vi "SetExternalInterface.vi"(8 "ErrorIn":errorcluster, 10 "ObjectName":string) -> (0 "ErrorOut":errorcluster)   [LabVIEW 2021]
uses:
  Interface_TAF_ITAFObject/ITAFObject/ITAFObject.lvclass
  Interface_TAF_IApplicationConfiguration/IApplicationConfiguration/IApplicationConfiguration.lvclass
  Application.lvclass
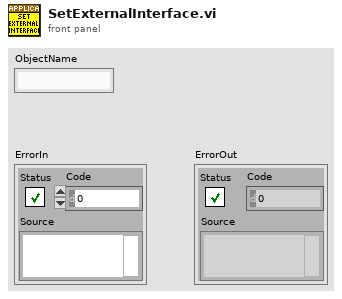
[diagram p1: front panel]
types:
  T1 = typedef "Application.lvclass/ObjectAttributes.ctl" = cluster{"Objects":variant, "BasePath":path, "Application":refnum<class "Application.lvclass">}
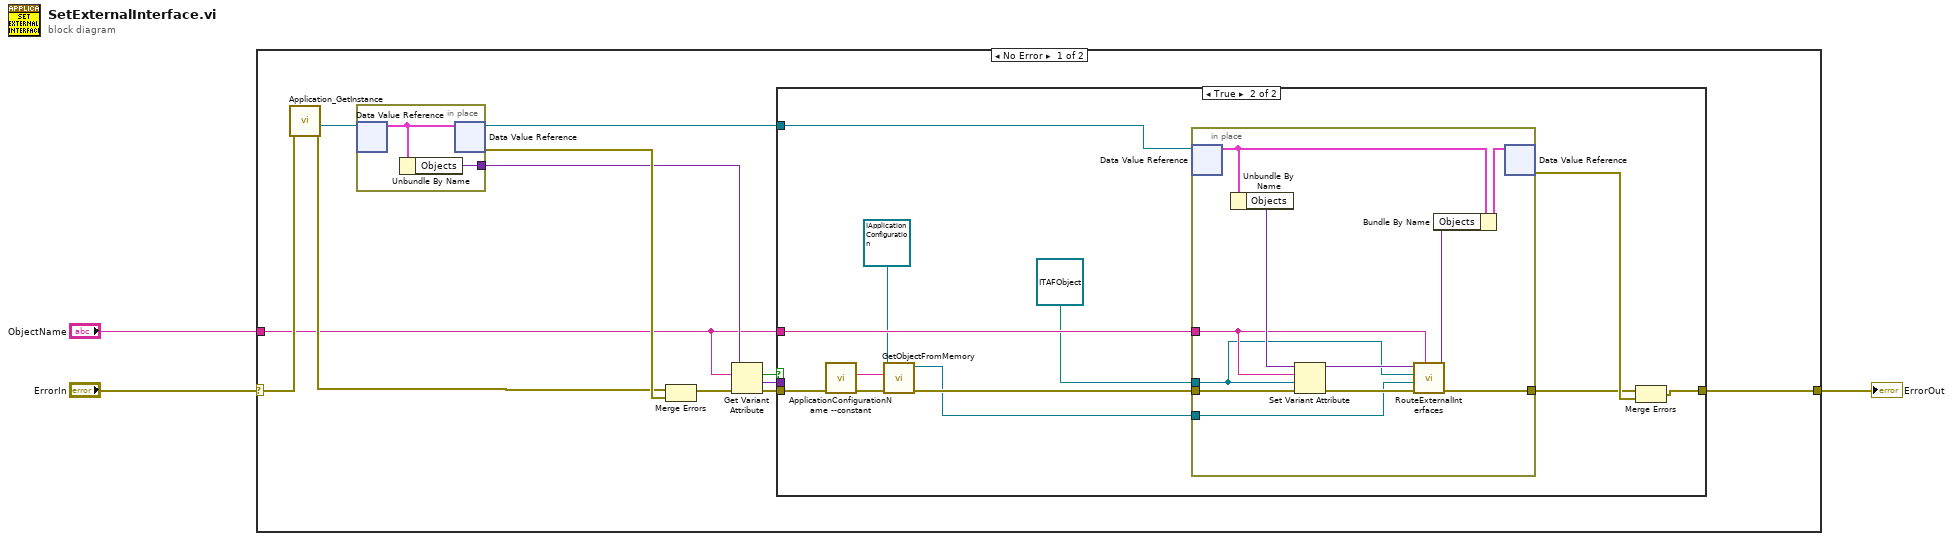
[diagram p0: block diagram]
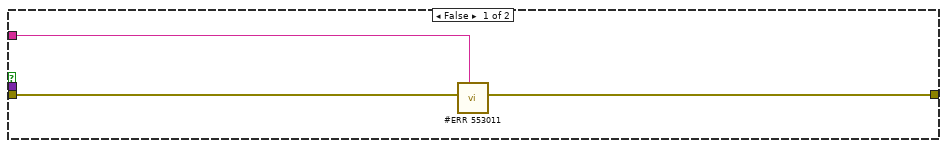
[diagram p2: hidden frame]
diagram:
  n1 = case shown="No Error" "ErrorIn" {
    selector: "ErrorIn" -> [w15 w43]
    tunnel: [w11 w43] -> w2
    tunnel: "ObjectName" -> [w4 _]
    frame No Error {
      n2 = call "Application_GetInstance.vi"("ErrorIn"=w15) -> ("ErrorOut"=w10:errorcluster, "DVRRefOut"=w9:refnum<data-value>)  [unwired: 6 in, 3 out]
      n3 = in-place {
        in-place-border: [w41] -> w6
        n4 = in-place-dvr #1(w9) -> (w42:T1)  [unwired: 1 out]
        n5 = Unbundle By Name(w42) -> ("Objects"=w41:variant)
        n6 = in-place-dvr #1(w42) -> (w5:refnum<data-value>, w14:errorcluster)
      }
      n7 = Merge Errors(w10, w14) -> (w13:errorcluster)
      n8 = Get Variant Attribute(Variant=w6, name=w4, error in=w13) -> (found=w8:bool, value=w7:variant, error out=w12:errorcluster)  [unwired: 1 in, 1 out]
      n9 = case shown="True" w8 {
        tunnel: w12 -> [w18 w26]
        tunnel: [w17 w29] -> w11
        tunnel: w7 -> [_ _]
        tunnel: w5 -> [_ w24]
        tunnel: w4 -> [w16 w23]
        frame False {
          n10 = call "#ERR 553011"("Data"=w16, "error in (no error)"=w18) -> ("error out"=w17:errorcluster)  [unwired: 9 in]
        }
        frame True {
          n11 = call "ApplicationConfigurationName --constant.vi"() -> ("AppConfigName"=w21:string)  [unwired: 10 in, 1 out]
          n12 = call "GetObjectFromMemory.vi"("ErrorIn"=w26, "ObjectName"=w21, "Type"=refnum<class "IApplicationConfiguration.lvclass"> refnum ("IApplicationStructure")) -> ("ErrorOut"=w25:errorcluster, "ObjectOut"=w20:refnum<class "IApplicationConfiguration.lvclass">)  [unwired: 7 in]
          n13 = in-place {
            in-place-border: w23 -> [w32]
            in-place-border: w25 -> [w40]
            in-place-border: [w39] -> w27
            in-place-border: w20 -> [w31]
            in-place-border: refnum<class "ITAFObject.lvclass"> refnum ("ClassActor") -> [w30]
            n14 = in-place-dvr #2(w24) -> (w37:T1)  [unwired: 1 out]
            n15 = Unbundle By Name(w37) -> ("Objects"=w35:variant)
            n16 = Set Variant Attribute(Variant=w35, name=w32, value=w30, error in=w40) -> (Variant out=w34:variant, error out=w38:errorcluster)  [unwired: 1 out]
            n17 = call "RouteExternalInterfaces.vi"("ObjectName"=w32, "ErrorIn"=w38, "ConfigObject"=w31, "ITAFObjectIn"=w30, "VariantIn"=w34) -> ("ErrorOut"=w39:errorcluster, "VariantOut"=w33:variant)  [unwired: 5 in]
            n18 = Bundle By Name(cluster=w37, "Objects"=w33) -> (w36:T1)
            n19 = in-place-dvr #2(w36) -> (w28:errorcluster)  [unwired: 1 out]
          }
          n20 = Merge Errors(w27, w28) -> (w29:errorcluster)
        }
      }
    }
    frame Error {
    }
  }
  "ErrorOut" <- w2
